vi "test_ram.vi"(0 "ram_address_in":u16, 1 "state_in":T1, 2 "data4inc_write_IN":u8) -> (7 "ram_address_out":u16, 8 "state_out":T1, 9 "data4inc_write_OUT":u8, 10 "ram_ok":bool)   [LabVIEW 2015]
uses:
  state_type.ctl
  <vilib>/rvi/eio/common/nirviEmuTemplateMethod_errors.vi
  <vilib>/eio/EIONode/EIONode.xnode
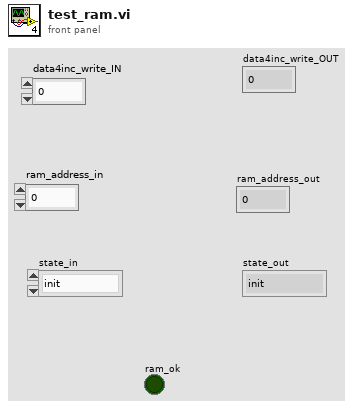
[diagram p1: front panel]
types:
  T1 = typedef "state_type.ctl" = enum16{"init", "write 0", "read 0", "write 1", "read 1", "write inc", "read inc"}
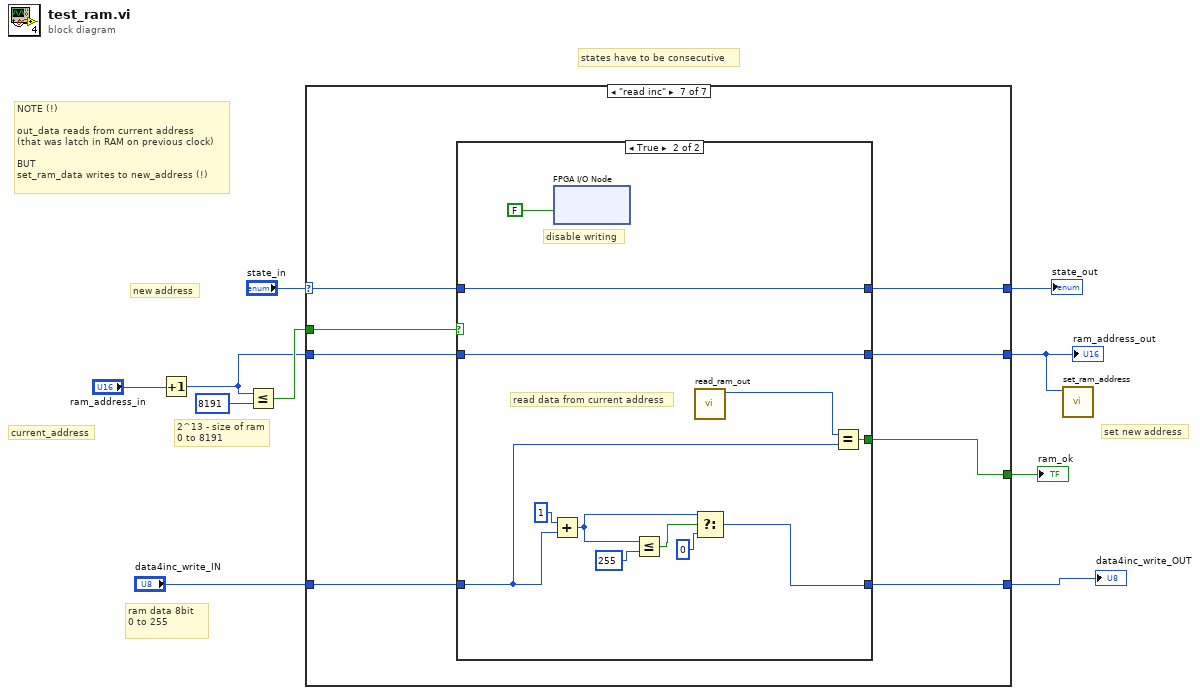
[diagram p0: block diagram]
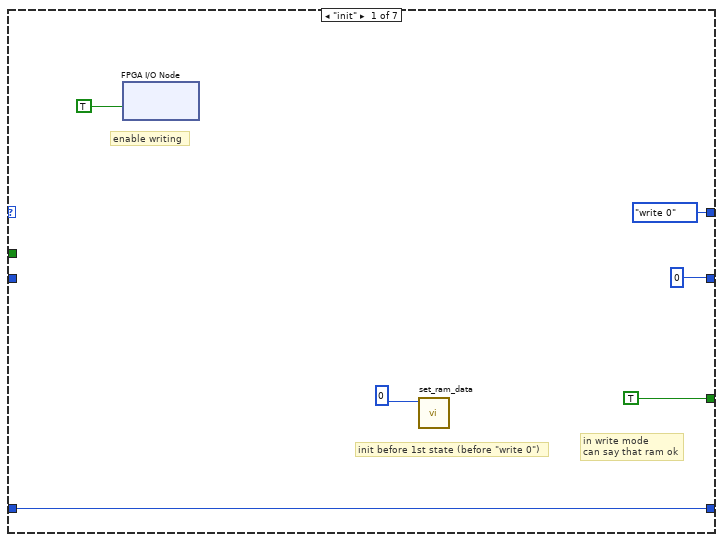
[diagram p2: hidden frame]
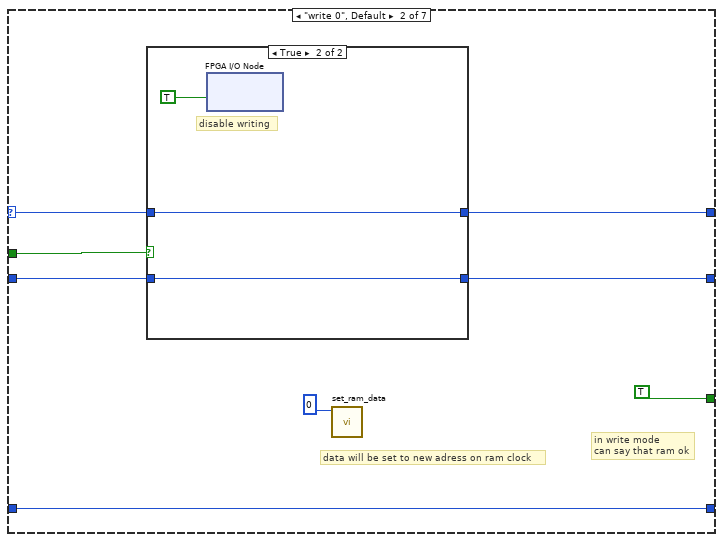
[diagram p3: hidden frame]
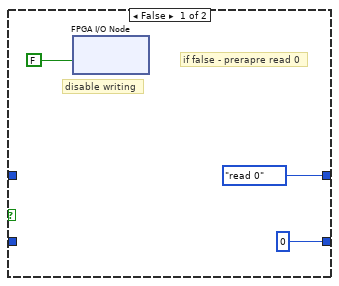
[diagram p4: hidden frame]
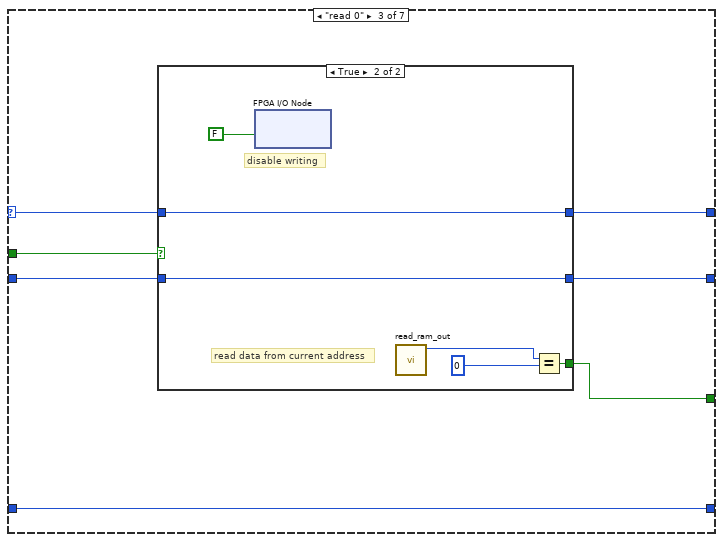
[diagram p5: hidden frame]
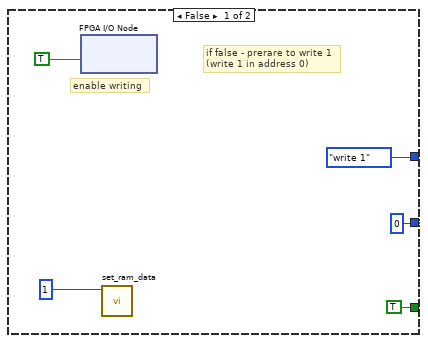
[diagram p6: hidden frame]
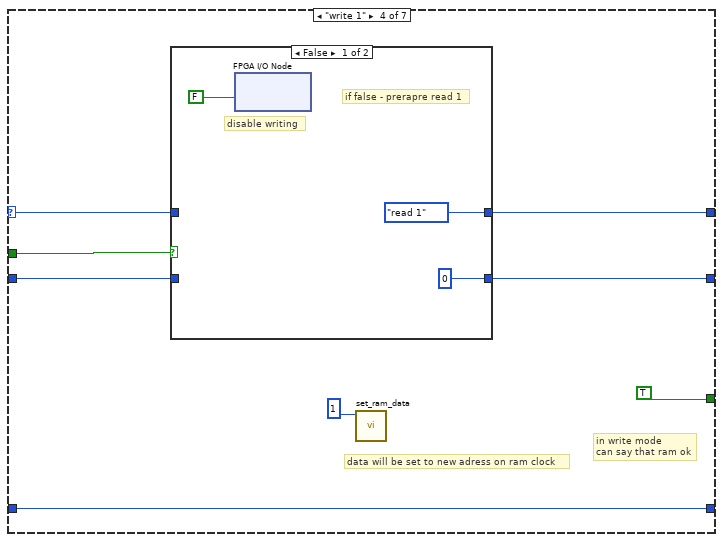
[diagram p7: hidden frame]
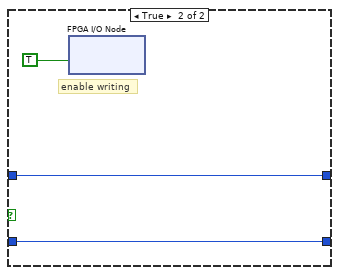
[diagram p8: hidden frame]
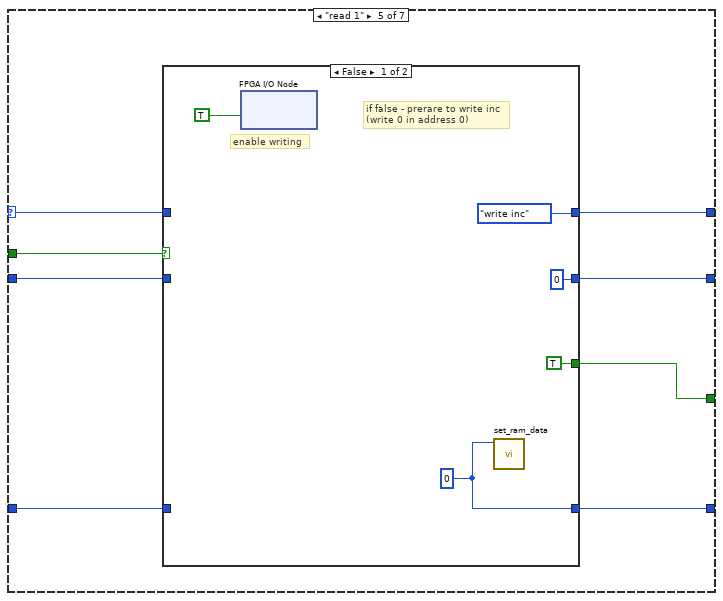
[diagram p9: hidden frame]
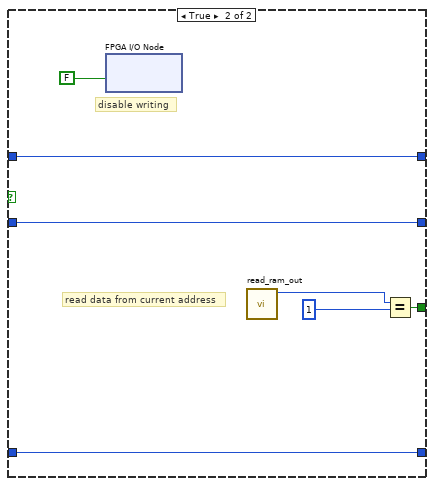
[diagram p10: hidden frame]
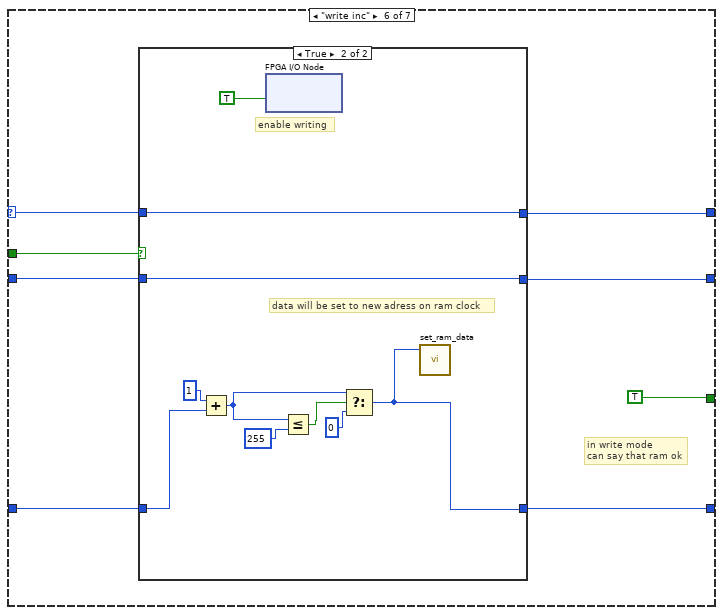
[diagram p11: hidden frame]
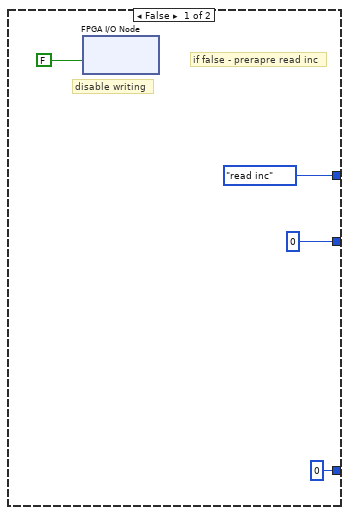
[diagram p12: hidden frame]
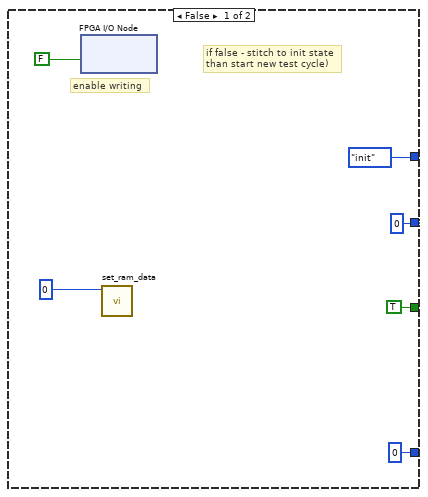
[diagram p13: hidden frame]
diagram:
  # "ram data 8bit\n0 to 255"
  # "set new address"
  # "NOTE (!)\n\nout_data reads from current address\n(that was latch in RAM on previous clock)\n\nBUT\nset_ram_data writes to new_address (!)"
  # "new address"
  # "current_address"
  # "states have to be consecutive"
  # "2^13 - size of ram\n0 to 8191"
  n1 = Increment(x="ram_address_in") -> (x+1=w7:u16)
  n2 = Less Or Equal?(x=w7, y=u16 8191 ("ram_adress 2")) -> (x <= y?=w8:bool)
  n3 = case shown="\"read inc\"" "state_in" {
    selector: "state_in" -> [_ w19 w35 w54 w66 w89 w112]
    tunnel: w8 -> [_ w20 w37 w52 w67 w90 w107]
    tunnel: w7 -> [_ w22 w36 w50 w68 w85 w108]
    tunnel: [u16 0 ("ram_adress") w21 w32 w51 w69 w87 w109] -> w4
    tunnel: [TRUE TRUE w33 TRUE w65 TRUE w110] -> w6
    tunnel: [state_type."write 0" ("f") w18 w34 w53 w70 w88 w111] -> w5
    tunnel: "data4inc_write_IN" -> [w11 w17 w31 w49 w64 w84 w106]
    tunnel: [w11 w17 w31 w49 w63 w83 w105] -> w1
    frame "init" {
      # "enable writing"
      # "in write mode\ncan say that ram ok"
      # "init before 1st state (before \"write 0\")"
      n4 = xnode "FPGA I/O Node"("we"=TRUE) -> ()  [unwired: 1 in, 1 out]
      n5 = call "set_ram_data.vi"("ram_data"=u8 0) -> ()  [unwired: 11 in]
    }
    frame "write 0", Default {
      # "data will be set to new adress on ram clock"
      # "in write mode\ncan say that ram ok"
      n6 = case shown="True" w20 {
        tunnel: w22 -> [_ w29]
        tunnel: [u16 0 ("f") w29] -> w21
        tunnel: w19 -> [_ w28]
        tunnel: [state_type."read 0" ("f") w28] -> w18
        frame False {
          # "if false - prerapre read 0"
          # "disable writing"
          n7 = xnode "FPGA I/O Node"("we"=FALSE) -> ()  [unwired: 1 in, 1 out]
        }
        frame True {
          # "disable writing"
          n8 = xnode "FPGA I/O Node"("we"=TRUE) -> ()  [unwired: 1 in, 1 out]
        }
      }
      n9 = call "set_ram_data.vi"("ram_data"=u8 0) -> ()  [unwired: 11 in]
    }
    frame "read 0" {
      n10 = case shown="True" w37 {
        tunnel: [u16 0 ("f") w47] -> w32
        tunnel: w36 -> [_ w47]
        tunnel: w35 -> [_ w43]
        tunnel: [state_type."write 1" ("f") w43] -> w34
        tunnel: [TRUE w46] -> w33
        frame False {
          # "if false - prerare to write 1\n(write 1 in address 0)"
          # "enable writing"
          n11 = xnode "FPGA I/O Node"("we"=TRUE) -> ()  [unwired: 1 in, 1 out]
          n12 = call "set_ram_data.vi"("ram_data"=u8 1) -> ()  [unwired: 11 in]
        }
        frame True {
          # "read data from current address"
          # "disable writing"
          n13 = xnode "FPGA I/O Node"("we"=FALSE) -> ()  [unwired: 1 in, 1 out]
          n14 = call "read_ram_out.vi"() -> ("RAM_OUT"=w44:u8)  [unwired: 11 in]
          n15 = Equal?(x=w44, y=u8 0 ("x")) -> (x = y?=w46:bool)
        }
      }
    }
    frame "write 1" {
      # "data will be set to new adress on ram clock"
      # "in write mode\ncan say that ram ok"
      n16 = case shown="False" w52 {
        tunnel: [u16 0 ("f") w60] -> w51
        tunnel: w54 -> [_ w61]
        tunnel: [state_type."read 1" ("f") w61] -> w53
        tunnel: w50 -> [_ w60]
        frame False {
          # "if false - prerapre read 1"
          # "disable writing"
          n17 = xnode "FPGA I/O Node"("we"=FALSE) -> ()  [unwired: 1 in, 1 out]
        }
        frame True {
          # "enable writing"
          n18 = xnode "FPGA I/O Node"("we"=TRUE) -> ()  [unwired: 1 in, 1 out]
        }
      }
      n19 = call "set_ram_data.vi"("ram_data"=u8 1) -> ()  [unwired: 11 in]
    }
    frame "read 1" {
      n20 = case shown="False" w67 {
        tunnel: [u16 0 ("f") w81] -> w69
        tunnel: w68 -> [_ w81]
        tunnel: w66 -> [_ w77]
        tunnel: [state_type."write inc" ("f") w77] -> w70
        tunnel: [TRUE w80] -> w65
        tunnel: w64 -> [_ w76]
        tunnel: [w71 w76] -> w63
        frame False {
          w71 = u8 0 ("ram_data")
          # "if false - prerare to write inc\n(write 0 in address 0)"
          # "enable writing"
          n21 = xnode "FPGA I/O Node"("we"=TRUE) -> ()  [unwired: 1 in, 1 out]
          n22 = call "set_ram_data.vi"("ram_data"=w71) -> ()  [unwired: 11 in]
        }
        frame True {
          # "read data from current address"
          # "disable writing"
          n23 = xnode "FPGA I/O Node"("we"=FALSE) -> ()  [unwired: 1 in, 1 out]
          n24 = call "read_ram_out.vi"() -> ("RAM_OUT"=w78:u8)  [unwired: 11 in]
          n25 = Equal?(x=w78, y=u8 1 ("x")) -> (x = y?=w80:bool)
        }
      }
    }
    frame "write inc" {
      # "in write mode\ncan say that ram ok"
      n26 = case shown="True" w90 {
        tunnel: [u16 0 ("f") w102] -> w87
        tunnel: [state_type."read inc" ("f") w103] -> w88
        tunnel: w89 -> [_ w103]
        tunnel: w85 -> [_ w102]
        tunnel: w84 -> [_ w101]
        tunnel: [u8 0 ("f") w95] -> w83
        frame False {
          # "if false - prerapre read inc"
          # "disable writing"
          n27 = xnode "FPGA I/O Node"("we"=FALSE) -> ()  [unwired: 1 in, 1 out]
        }
        frame True {
          # "data will be set to new adress on ram clock"
          # "enable writing"
          n28 = Add(x=u8 1, y=w101) -> (x+y=w97:u8)
          n29 = xnode "FPGA I/O Node"("we"=TRUE) -> ()  [unwired: 1 in, 1 out]
          n30 = Less Or Equal?(x=w97, y=u8 255) -> (x <= y?=w98:bool)
          n31 = Select(t=w97, s=w98, f=u8 0) -> (s? t:f=w95:u8)
          n32 = call "set_ram_data.vi"("ram_data"=w95) -> ()  [unwired: 11 in]
        }
      }
    }
    frame "read inc" {
      n33 = case shown="True" w107 {
        tunnel: [u16 0 ("f") w126] -> w109
        tunnel: w112 -> [_ w127]
        tunnel: [state_type."init" ("f") w127] -> w111
        tunnel: [TRUE w129] -> w110
        tunnel: w108 -> [_ w126]
        tunnel: w106 -> [_ w120]
        tunnel: [u8 0 ("data4inc_write_IN") w119] -> w105
        frame False {
          # "if false - stitch to init state\nthan start new test cycle)"
          # "enable writing"
          n34 = xnode "FPGA I/O Node"("we"=FALSE) -> ()  [unwired: 1 in, 1 out]
          n35 = call "set_ram_data.vi"("ram_data"=u8 0) -> ()  [unwired: 11 in]
        }
        frame True {
          # "read data from current address"
          # "disable writing"
          n36 = Add(x=u8 1, y=w120) -> (x+y=w122:u8)
          n37 = xnode "FPGA I/O Node"("we"=FALSE) -> ()  [unwired: 1 in, 1 out]
          n38 = Less Or Equal?(x=w122, y=u8 255) -> (x <= y?=w123:bool)
          n39 = call "read_ram_out.vi"() -> ("RAM_OUT"=w128:u8)  [unwired: 11 in]
          n40 = Select(t=w122, s=w123, f=u8 0) -> (s? t:f=w119:u8)
          n41 = Equal?(x=w128, y=w120) -> (x = y?=w129:bool)
        }
      }
    }
  }
  "ram_address_out" <- w4
  "ram_ok" <- w6
  "state_out" <- w5
  "data4inc_write_OUT" <- w1
  n42 = call "set_ram_address.vi"("ram_adress"=w4) -> ()  [unwired: 11 in]
